vi "Untitled 2.vi"   [LabVIEW 2023]
uses:
  <vilib>/Platform/storage/lvStorage.llb/xStorage/Write Data/Write Data.xnode
  <vilib>/Platform/storage/Storage.llb/usiSequenceRepresentation.ctl
  <vilib>/Platform/storage/Storage.llb/usiOverwriteOptions.ctl
  <vilib>/Platform/storage/lvStorage.llb/_createOrGetByNameExplicitChildObject.vi
  <vilib>/Platform/storage/lvStorage.llb/_getChannelNameFromDDT.vi
  <vilib>/Platform/storage/lvStorage.llb/_saveDDT.vi
  <vilib>/Platform/storage/Storage.llb/__savePropString.vi
  <vilib>/Platform/storage/lvStorage.llb/_prepDDT.vi
  <vilib>/Platform/storage/lvStorage.llb/xStorage/xStorageSupp/ErrorOut.vi
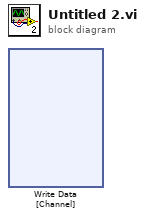
[diagram p0: block diagram]
diagram:
  n1 = xnode "Write Data\n[Channel]"() -> ()  [unwired: 6 in, 3 out]
